vi "Image_Save_Handler.vi"(0 "first iteration":bool, 4 "Data":T3={"system"={"info"={"menuSelect"=0, "version"=0, "serial"="Test Sample", "captureActive"=FALSE, "captureBegin"=FALSE, "emptyAndRefill"=FALSE}, "userInfo"={"operatorName"="", "date"=timestamp(2713993200 s since 1904-01-01)}, "camera"={"exposureTime"=0, "aperture"=enum."Item 0", "framerate"=0, "framerateMax"=500, "legacyAttributes"=FALSE}}, "connections"={"arduino"={"connection"="MRJ", "status"=FALSE, "openState"=FALSE, "emptyStart"=0}, "pump"={"connection"="MRJ", "status"=FALSE, "command"="", "dispenseSpeed"=100, "flushSize"=100}, "camera"={"cam1"={"connection"="", "status"=FALSE}, "cam2"={"connection"="", "status"=FALSE}}}, "queue"={"process"={"cam1"=refnum, "cam2"=refnum, "queueSize"=0}, "save"={"cam1"=refnum, "cam2"=refnum, "queueSize"=0}, "overloadThreshold"=0}, "imageProcess"={"cam1"={"preAllocation"={"image"="Station", "originalDisplay"="Station", "originalRgb"="Station", "binary"="Station", "save"="Station", "calibrationFull"=refnum, "calibrationDetect"=refnum}, "calibration"={"pathFull"=path "C:/Users/au540322/Desktop/IHS_Project/images/Debris/Debris_0/Debris_0_2019_06_01-23-32-49-686.PNG", "pathDetect"=path "C:/Users/au540322/Desktop/IHS_Project/images/Debris/Debris_0/Debris_0_2019_06_01-23-32-49-686.PNG", "ROI"={"Left"=0, "Top"=0, "Right"=0, "Bottom"=0, "Rotation"=0.0}}}, "cam2"={"preAllocation"={"image"=refnum, "originalDisplay"=refnum, "originalRgb"=refnum, "binary"=refnum, "save"=refnum, "calibrationFull"=refnum, "calibrationDetect"=refnum}, "calibration"={"pathFull"=path "C:/Users/au540322/Desktop/IHS_Project/images/Debris/Debris_0/Debris_0_2019_06_01-23-32-49-686.PNG", "pathDetect"=path "C:/Users/au540322/Desktop/IHS_Project/images/Debris/Debris_0/Debris_0_2019_06_01-23-32-49-686.PNG", "ROI"={"Left"=0, "Top"=0, "Right"=0, "Bottom"=0, "Rotation"=0.0}}}, "process"={"planeExtract"=refnum, "planeSubtract"=refnum, "cropMask"=refnum}, "detection"={"sampleTimeout"=500, "sizeThreshold"=500, "detectionRegionPct"=0.0}}, "sampleData"={"sampleId"="", "projectId"="", "voucherID"="", "speciesName"="", "collectionDate"=timestamp(2713993200 s since 1904-01-01), "sampleStation"="", "location"="", "lat"=0.0, "lon"=0.0, "determiner"="", "sex"="", "otherNotes"=""}, "Session In"=""} {"sampleData"."collectionDate" format="%<%Y-%m-%d>T"; "imageProcess"."detection"."sizeThreshold" min=1; "imageProcess"."cam2"."calibration"."ROI"."Rotation" format="%.2f"; "imageProcess"."cam2"."calibration"."ROI"."Left" scale=0.0..1024.0; "imageProcess"."cam2"."calibration"."ROI"."Right" scale=0.0..1024.0; "imageProcess"."cam1"."calibration"."ROI"."Rotation" format="%.2f"; "imageProcess"."cam1"."calibration"."ROI"."Left" scale=0.0..1024.0; "imageProcess"."cam1"."calibration"."ROI"."Right" scale=0.0..1024.0; "queue"."overloadThreshold" min=1; "queue"."save"."queueSize" min=1; "queue"."process"."queueSize" min=1; "connections"."pump"."flushSize" min=1; "connections"."pump"."dispenseSpeed" min=1; "system"."camera"."framerateMax" min=1; "system"."userInfo"."date" format="%<%Y-%m-%dT%H:%M:%S+%z>T"; "system"."info"."version" items=["Standard", "XL"]; "system"."info"."menuSelect" items=["Session Data", "Extended Setup", "Buffer", "Camera", "Dispenser", "Stats", "Connections"]}, 7 "Stop?":bool) -> (12 "Image Save 1":T1, 14 "Image Save 2":T1, 17 "Cam2_Stats":cluster{"Mean_Area":i32, "Img_Count":u32} caption="Camera 2", 19 "Cam1_Stats":cluster{"Mean_Area":i32, "Img_Count":u32} caption="Camera 1", 20 "Queue size":T2, 23 "timeout":bool, 24 "max queue":i32, 25 "Sample Name":string, 27 "Stop out":bool)   [LabVIEW 2022 SP3]
doc: "Saves image files from cameras in specified folder location."
uses:
  controls/Data.ctl
  <vilib>/userdefined/High Color/IMAQdx.ctl
  <vilib>/vision/Image Controls.llb/IMAQ Image.ctl
  Camera_ID.ctl
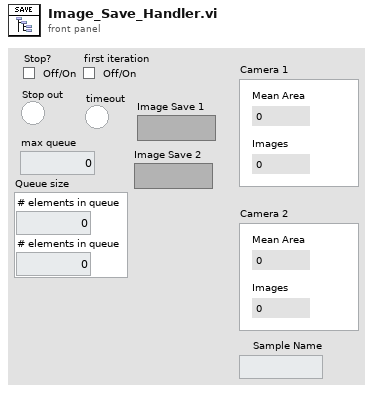
[diagram p1: front panel]
types:
  T1 = typedef "IMAQ Image.ctl" = refnum<image>
  T2 = cluster{"# elements in queue":i32, "# elements in queue":i32}
  T3 = typedef "Data.ctl" = cluster{"system":cluster{"info":cluster{"menuSelect":u16, "version":u16, "serial":string, "captureActive":bool, "captureBegin":bool, "emptyAndRefill":bool}, "userInfo":cluster{"operatorName":string, "date":timestamp}, "camera":cluster{"exposureTime":i32, "aperture":enum32{"Item 0", "Item 1", "Item 2", "Item 3"}, "framerate":i32, "framerateMax":i32, "legacyAttributes":bool}}, "connections":cluster{"arduino":cluster{"connection":refnum<visa-resource-name>, "status":bool, "openState":bool, "emptyStart":u32}, "pump":cluster{"connection":refnum<visa-resource-name>, "status":bool, "command":string, "dispenseSpeed":i32, "flushSize":i32}, "camera":cluster{"cam1":cluster{"connection":T4, "status":bool}, "cam2":cluster{"connection":T4, "status":bool}}}, "queue":cluster{"process":cluster{"cam1":refnum<queue>, "cam2":refnum<queue>, "queueSize":i32}, "save":cluster{"cam1":refnum<queue>, "cam2":refnum<queue>, "queueSize":i32}, "overloadThreshold":i32}, "imageProcess":cluster{"cam1":cluster{"preAllocation":cluster{"image":T1, "originalDisplay":T1, "originalRgb":T1, "binary":T1, "save":T1, "calibrationFull":T1, "calibrationDetect":T1}, "calibration":cluster{"pathFull":path, "pathDetect":path, "ROI":T5}}, "cam2":cluster{"preAllocation":cluster{"image":T1, "originalDisplay":T1, "originalRgb":T1, "binary":T1, "save":T1, "calibrationFull":T1, "calibrationDetect":T1}, "calibration":cluster{"pathFull":path, "pathDetect":path, "ROI":T5}}, "process":cluster{"planeExtract":T1, "planeSubtract":T1, "cropMask":T1}, "detection":cluster{"sampleTimeout":i32, "sizeThreshold":i32, "detectionRegionPct":dbl}}, "sampleData":cluster{"sampleId":string, "projectId":string, "voucherID":string, "speciesName":string, "collectionDate":timestamp, "sampleStation":string, "location":string, "lat":dbl, "lon":dbl, "determiner":string, "sex":string, "otherNotes":string}, "Session In":T4}
  T4 = typedef "IMAQdx.ctl" = refnum<k21>
  T5 = typedef "IMAQ Rectangle" = cluster{"Left":i32, "Top":i32, "Right":i32, "Bottom":i32, "Rotation":dbl}
  T6 = typedef "Camera_ID.ctl" = enum16{"Camera 1", "Camera 2"}
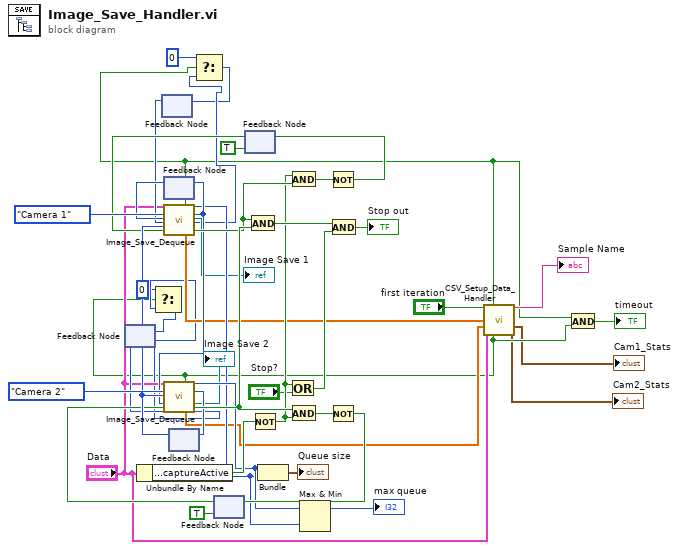
[diagram p0: block diagram]
diagram:
  n1 = feedback #1() -> (w12:u32)  [unwired: 1 in]
  n2 = Unbundle By Name("Data") -> ("system.info.captureActive"=w41:bool)
  n3 = feedback #2() -> (w13:u32)  [unwired: 1 in]
  n4 = feedback #3() -> (w34:i32)  [unwired: 1 in]
  n5 = feedback #4() -> (w32:i32)  [unwired: 1 in]
  n6 = feedback #5(TRUE) -> (w27:bool)
  n7 = feedback #6(TRUE) -> (w29:bool)
  n8 = call "Image_Save_Dequeue.vi"("Data"="Data", "Camera"=Camera_ID."Camera 1", "Old"=w34, "cam1_prev"=w13, "Other"=w32, "Queue active"=w29) -> ("timed out?"=w4:bool, "Sample Data"=w14:dbl[], "# elements in queue"=w22:i32, "State out"=w31:i32, "Image Save 1"=→"Image Save 1":T1, "cam1_count"=w10:u32, "Last image"=w38:bool)  [unwired: 13 in, 2 out]
  n9 = feedback-in #3(w31) -> ()
  n10 = call "Image_Save_Dequeue.vi"("Data"="Data", "Camera"=Camera_ID."Camera 2", "Old"=w32, "Other"=w31, "Queue active"=w27, "cam2_prev"=w12) -> ("timed out?"=w3:bool, "Sample Data"=w20:dbl[], "# elements in queue"=w23:i32, "State out"=w33:i32, "Image Save 2"=→"Image Save 2":T1, "Last image"=w40:bool, "cam2_count"=w6:u32)  [unwired: 13 in, 2 out]
  n11 = Select(t=u32 0, s=w3, f=w6) -> (s? t:f=w7:u32)
  n12 = feedback-in #1(w7) -> ()
  n13 = feedback-in #4(w33) -> ()
  n14 = Select(t=u32 0, s=w4, f=w10) -> (s? t:f=w9:u32)
  n15 = feedback-in #2(w9) -> ()
  n16 = And(x=w38, y=w40) -> (x .and. y?=w44:bool)
  n17 = Not(x=w41) -> (.not. x?=w37:bool)
  n18 = Bundle("# elements in queue"=w23, "# elements in queue"=w22) -> (→"Queue size":T2)  [unwired: 1 in]
  n19 = Or(x=w37, y="Stop?") -> (x .or. y?=w42:bool)
  n20 = And(x=w37, y=w38) -> (x .and. y?=w36:bool)
  n21 = And(x=w40, y=w37) -> (x .and. y?=w39:bool)
  n22 = Max & Min(x=w23, y=w22) -> (max(x,y)=→"max queue":i32)  [unwired: 1 out]
  n23 = Not(x=w36) -> (.not. x?=w30:bool)
  n24 = feedback-in #6(w30) -> ()
  n25 = Not(x=w39) -> (.not. x?=w28:bool)
  n26 = feedback-in #5(w28) -> ()
  n27 = And(x=w44, y=w42) -> (x .and. y?=→"Stop out":bool)
  n28 = call "CSV_Setup_Data_Handler.vi"("first iteration"="first iteration", "Timeout 1"=w4, "Sample Data"=w14, "Sample Data 2"=w20, "Data"="Data", "Timeout 2"=w3) -> ("Sample Name"=→"Sample Name":string, "Cam1_Stats"=→"Cam1_Stats":cluster{"Mean_Area":i32, "Img_Count":u32}, "Cam2_Stats"=→"Cam2_Stats":cluster{"Mean_Area":i32, "Img_Count":u32})  [unwired: 7 in]
  n29 = And(x=w4, y=w3) -> (x .and. y?=→"timeout":bool)
